vi "SDSU_SetCmdAdd.vi"(8 "error in (no error)":errorcluster, 10 "translations path":path=path "/home/bonati/PAN/Modules/MNSN/private/c/test/command_translations.cfg") -> (0 "error out":errorcluster, 2 "Array":T1[](array[typedef]))   [LabVIEW 2016]
uses:
  SDSU_cmdTableEntry.ctl
  <vilib>/Utility/config.llb/Read Key (String).vi
  <vilib>/Utility/config.llb/NI_LVConfig.lvlib
panel:
  out "translations path 2":path=path "/home/bonati/PAN/Modules/MNSN/private/c/test/command_translations.cfg"
  in  "Cluster":T1
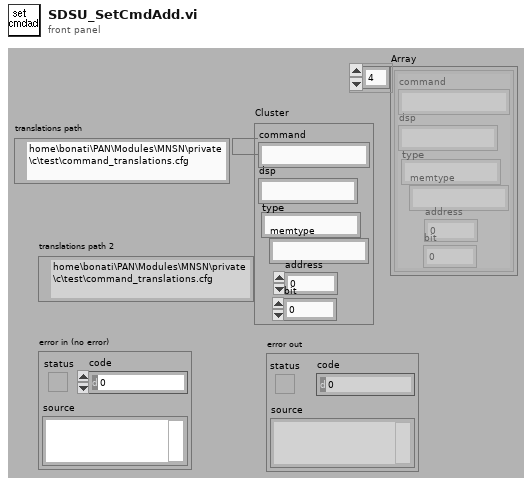
[diagram p1: front panel]
types:
  T1 = typedef "SDSU_cmdTableEntry.ctl" = cluster{"command":string, "dsp":string, "type":string, "memtype":string, "address":i32, "bit":i32}
  T2 = typedef "NI_LVConfig.lvlib/Config Data RefNum.ctl" = refnum<k1>
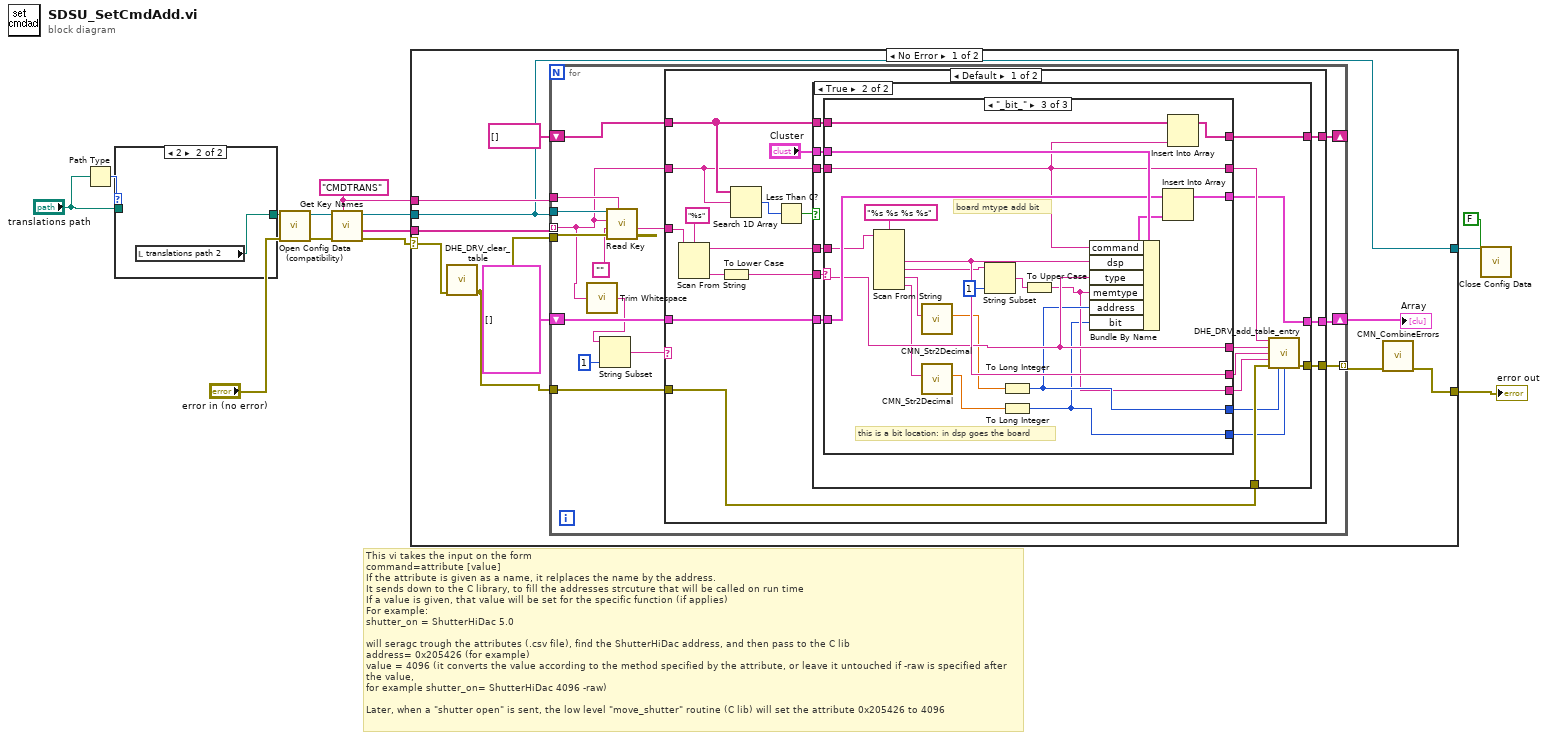
[diagram p0: block diagram]
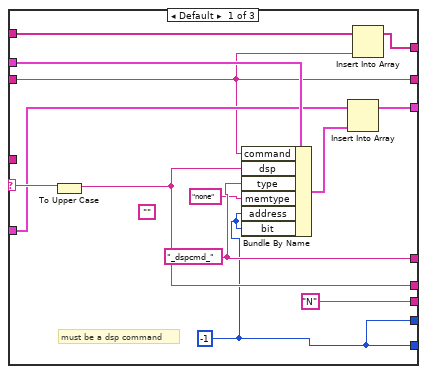
[diagram p3: hidden frame]
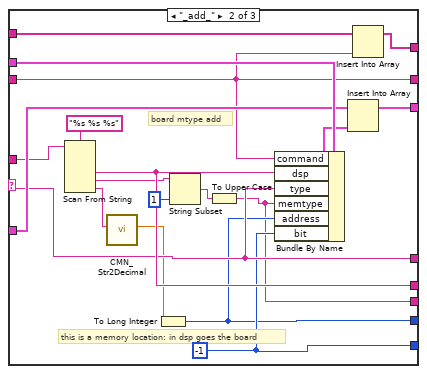
[diagram p4: hidden frame]
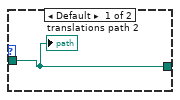
[diagram p7: hidden frame]
diagram:
  w9 = "CMDTRANS" ("section")
  # "This vi takes the input on the form\ncommand=attribute [value]\nIf the attribute is given as a name, it relplaces the name by the address.\nIt sends down to the C library, to fill the addresses strcuture that will be called on run time\nIf a value is given, that value will be set for the specific function (if applies)\nFor example:\nshutter_on = ShutterHiDac 5.0\n\nwill seragc trough the attributes (.csv file), find the ShutterHiDac address, and then pass to the C lib\naddress= 0x205426 (for example)\nvalue = 4096 (it converts the value according to the method specified by the attribute, or leave it untouched if -raw is specified after the value,\nfor example shutter_on= ShutterHiDac 4096 -raw)\n\nLater, when a \"shutter open\" is sent, the low level \"move_shutter\" routine (C lib) will set the attribute 0x205426 to 4096"
  n1 = Path Type(1:"translations path") -> (0:w7:i16)
  n2 = case shown="2" w7 {
    tunnel: "translations path" -> [w14 _]
    tunnel: [w14 w15] -> w5
    frame Default {
      "translations path 2" <- w14
    }
    frame 2 {
      n3 = local read "translations path 2"() -> (w15:path)
    }
  }
  n4 = call <vilib>:"Open Config Data (compatibility).vi"("error in (no error)"="error in (no error)", "configuration file path"=w5) -> ("error out"=w13:errorcluster, "refnum"=w12:T2)  [unwired: 7 in, 1 out]
  n5 = call <vilib>:"Get Key Names.vi"("section"=w9, "error in (no error)"=w13, "refnum"=w12) -> ("error out"=w3:errorcluster, "key names"=w11:string[], "refnum out"=w10:T2)  [unwired: 6 out]
  n6 = case shown="No Error" w3 {
    selector: w3 -> [w23 w132]
    tunnel: w11 -> [w25 _]
    tunnel: w10 -> [w22 w131]
    tunnel: w9 -> [w24 _]
    tunnel: [w19 w132] -> w4
    tunnel: [w22 w131] -> w2
    frame No Error {
      n7 = call "DHE_DRV_clear_table.vi"("error in (no error)"=w23) -> ("error out"=w21:errorcluster)  [unwired: 14 out]
      n8 = for {
        tunnel: w25 -> [w28] mode=indexing
        tunnel: w22 -> [w40]
        tunnel: w21 -> [w39]
        tunnel: w24 -> [w38]
        shift-right: [w36] -> w16
        shift-left: T1[] [] -> [w35]
        tunnel: w21 -> [w34]
        tunnel: [w33] -> w20 mode=indexing
        shift-right: [w27] -> _
        shift-left: string[] [] -> [w26]
        n9 = call <vilib>:"Trim Whitespace.vi"("string"=w28) -> ("trimmed string"=w31:string)  [unwired: 1 in]
        n10 = String Subset(string=w31, length (rest)=1 ("length (rest)")) -> (substring=w29:string)  [unwired: 1 out]
        n11 = call-poly <vilib>:"Read Key.vi"("section"=w38, "error in (no error)"=w39, "default value"="", "key"=w28, "refnum"=w40) -> ("value"=w32:string)  [unwired: 1 in, 5 out]
        n12 = case shown="Default" w29 {
          tunnel: w28 -> [w43 _]
          tunnel: [w46 w130] -> w36
          tunnel: w35 -> [w55 w130]
          tunnel: w32 -> [w52 _]
          tunnel: w34 -> [w50 w129]
          tunnel: [w49 w129] -> w33
          tunnel: [w45 w128] -> w27
          tunnel: w26 -> [w44 w128]
          frame Default {
            n13 = Scan From String(format string="%s", input string=w52) -> (remaining string=w51:string, output 1=w48:string)  [unwired: 2 in, 3 out]
            n14 = To Lower Case(string=w48) -> (all lower case string=w47:string)
            n15 = Search 1D Array(1D array=w44, element=w43) -> (index of element=w42:i32)  [unwired: 1 out]
            n16 = Less Than 0?(x=w42) -> (x < 0?=w41:bool)
            n17 = case shown="True" w41 {
              tunnel: w55 -> [w57 w74]
              tunnel: "Cluster" -> [_ w73]
              tunnel: w51 -> [_ w72]
              tunnel: w50 -> [w56 w71]
              tunnel: [w56 w70] -> w49
              tunnel: w47 -> [_ w67]
              tunnel: [w57 w62] -> w46
              tunnel: [w58 w61] -> w45
              tunnel: w44 -> [w58 w60]
              tunnel: w43 -> [_ w59]
              frame False {
                # "already added, skip"
              }
              frame True {
                n18 = case shown="\"_bit_\"" w67 {
                  selector: w67 -> [w87 w93 w114]
                  tunnel: w59 -> [w78 w102 w123]
                  tunnel: w74 -> [w81 w105 w126]
                  tunnel: w73 -> [w85 w106 w127]
                  tunnel: w72 -> [_ w99 w120]
                  tunnel: [w78 w102 w123] -> w69
                  tunnel: [w83 w93 w114] -> w68
                  tunnel: [w84 w97 w118] -> w66
                  tunnel: ["N" ("memtype") w88 w110] -> w65
                  tunnel: [w75 w89 w111] -> w64
                  tunnel: [w75 w90 w107] -> w63
                  tunnel: [w79 w103 w124] -> w62
                  tunnel: [w77 w101 w122] -> w61
                  tunnel: w60 -> [w76 w100 w121]
                  frame Default {
                    (unwired) ""
                    w75 = -1 ("bit")
                    w83 = "_dspcmd_" ("type")
                    # "must be a dsp command"
                    n19 = To Upper Case(1:w87) -> (0:w84:string)
                    n20 = Bundle By Name(cluster=w85, "command"=w78, "dsp"=w84, "type"=w83, "memtype"="none", "address"=w75, "bit"=w75) -> (w80:T1)
                    n21 = Insert Into Array(array=w81, new element=w80) -> (w79:T1[])  [unwired: 1 in]
                    n22 = Insert Into Array(array=w76, new element=w78) -> (w77:string[])  [unwired: 1 in]
                  }
                  frame "_add_" {
                    w90 = -1 ("bit")
                    # "board mtype add"
                    # "this is a memory location: in dsp goes the board"
                    n23 = Scan From String(format string="%s %s %s", input string=w99) -> (output 1=w97:string, output 2=w96:string, output 3=w92:string)  [unwired: 2 in, 6 out]
                    n24 = call "CMN_Str2Decimal.vi"("number in"=w92) -> ("decimal number"=w91:dbl)  [unwired: 1 in, 9 out]
                    n25 = To Long Integer(number=w91) -> (32bit integer=w89:i32)
                    n26 = String Subset(string=w96, length (rest)=1 ("length (rest)")) -> (substring=w94:string)  [unwired: 1 out]
                    n27 = To Upper Case(1:w94) -> (0:w88:string)
                    n28 = Bundle By Name(cluster=w106, "command"=w102, "dsp"=w97, "type"=w93, "memtype"=w88, "address"=w89, "bit"=w90) -> (w104:T1)
                    n29 = Insert Into Array(array=w105, new element=w104) -> (w103:T1[])  [unwired: 1 in]
                    n30 = Insert Into Array(array=w100, new element=w102) -> (w101:string[])  [unwired: 1 in]
                  }
                  frame "_bit_" {
                    # "board mtype add bit"
                    # "this is a bit location: in dsp goes the board"
                    n31 = Scan From String(format string="%s %s %s %s", input string=w120) -> (output 1=w118:string, output 2=w117:string, output 3=w113:string, output 4=w109:string)  [unwired: 2 in, 7 out]
                    n32 = call "CMN_Str2Decimal.vi"("number in"=w113) -> ("decimal number"=w112:dbl)  [unwired: 1 in, 9 out]
                    n33 = call "CMN_Str2Decimal.vi"("number in"=w109) -> ("decimal number"=w108:dbl)  [unwired: 1 in, 9 out]
                    n34 = String Subset(string=w117, length (rest)=1 ("length (rest)")) -> (substring=w115:string)  [unwired: 1 out]
                    n35 = To Long Integer(number=w112) -> (32bit integer=w111:i32)
                    n36 = To Long Integer(number=w108) -> (32bit integer=w107:i32)
                    n37 = To Upper Case(1:w115) -> (0:w110:string)
                    n38 = Bundle By Name(cluster=w127, "command"=w123, "dsp"=w118, "type"=w114, "memtype"=w110, "address"=w111, "bit"=w107) -> (w125:T1)
                    n39 = Insert Into Array(array=w126, new element=w125) -> (w124:T1[])  [unwired: 1 in]
                    n40 = Insert Into Array(array=w121, new element=w123) -> (w122:string[])  [unwired: 1 in]
                  }
                }
                n41 = call "DHE_DRV_add_table_entry.vi"("cmd"=w69, "type"=w68, "dsp"=w66, "memtype"=w65, "error in (no error)"=w71, "address"=w64, "bit"=w63) -> ("error out"=w70:errorcluster)  [unwired: 8 out]
              }
            }
          }
          frame "#", "/", ";" {
            # "this is a comment, ignoe"
          }
        }
      }
      "Array" <- w16
      n42 = call "CMN_CombineErrors.vi"("Errors"=w20) -> ("error out"=w19:errorcluster)  [unwired: 10 out]
    }
    frame Error {
    }
  }
  "error out" <- w4
  n43 = call <vilib>:"Close Config Data.vi"("write file if changed (T)"=FALSE ("write configuration file? (T)"), "refnum"=w2) -> ()  [unwired: 1 in, 9 out]
